vi "KGN Get Limits.vi"(8 "Fehler (Eingang, kein Fehler)":errorcluster, 9 "Info Cluster":T1, 10 "VISA-Ressourcenname":refnum<visa-resource-name>, 11 "device (Eingang)":u32) -> (0 "Fehler (Ausgang)":errorcluster, 1 "Info Cluster out":T1, 2 "VISA-Ressourcenname out":refnum<visa-resource-name>, 3 "dup device (Ausgang)":u32, 4 "Limits Cluster out":cluster{"flow":dbl[], "temp":dbl[]}, 6 "Kommnados gesendet":string)   [LabVIEW 2020, in "Linearisierung v2.lvlib" / "Gasteiler.lvlib" / "HovaCAL_Interface.lvlib" / "KGN.lvlib" / "KGN GUI Get.lvlib"]
uses:
  KGN GUI Get.lvlib
  Controls/Info Cluster.ctl
  get/get.lvlib
  Controls/Controls.lvlib
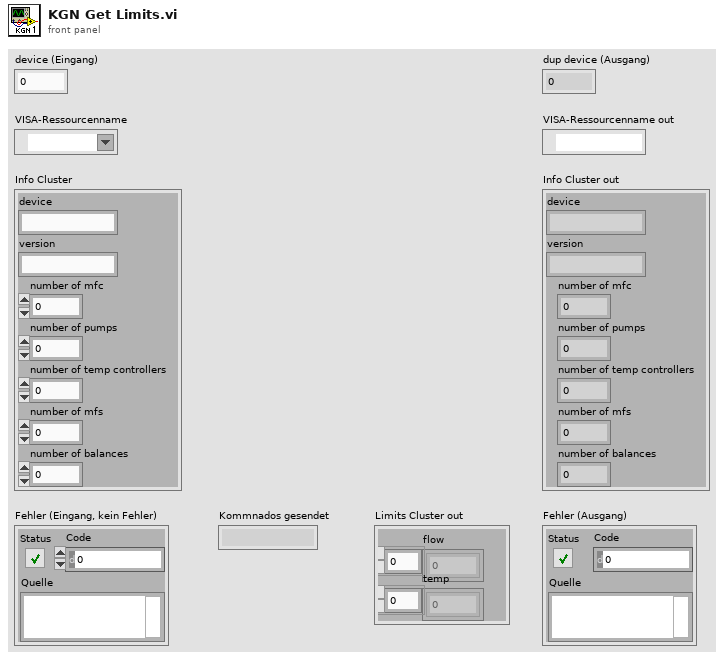
[diagram p1: front panel]
types:
  T1 = typedef "Linearisierung v2.lvlib/Gasteiler.lvlib/HovaCAL_Interface.lvlib/Controls.lvlib/Info Cluster.ctl" = cluster{"device":string, "version":string, "number of mfc":i32, "number of pumps":i32, "number of temp controllers":i32, "number of mfs":i32, "number of balances":i32}
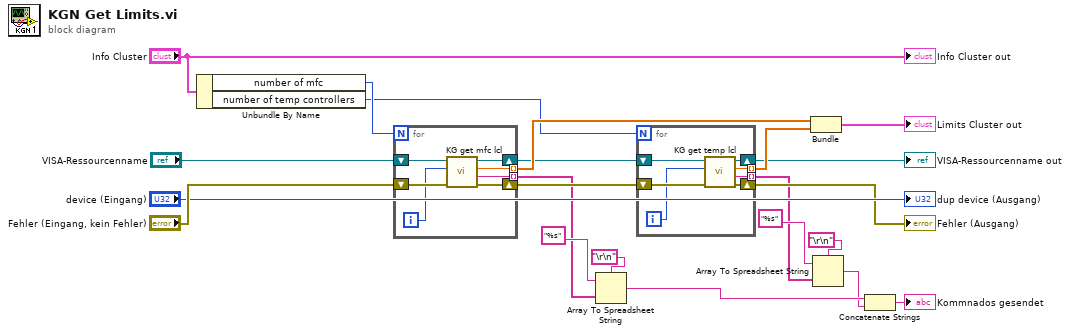
[diagram p0: block diagram]
diagram:
  n1 = Unbundle By Name("Info Cluster") -> ("number of mfc"=w11:i32, "number of temp controllers"=w10:i32)
  n2 = for {
    N: w11 -> [_]
    tunnel: [w28] -> w19 mode=indexing
    shift-right: [w25] -> w14
    shift-left: "Fehler (Eingang, kein Fehler)" -> [w29]
    shift-right: [w26] -> w17
    shift-left: "VISA-Ressourcenname" -> [w27]
    tunnel: [w23] -> w5 mode=indexing
    i -> [w24]
    n3 = call "KG get mfc lcl.vi"("Fehler (Eingang, kein Fehler)"=w29, "mfc"=w24, "VISA-Ressourcenname"=w27) -> ("Fehler (Ausgang)"=w25:errorcluster, "Kommando gesendet"=w23:string, "flow"=w28:dbl, "VISA-Ressourcenname (Ausgang)"=w26:refnum<visa-resource-name>)  [unwired: 5 in]
  }
  n4 = Array To Spreadsheet String(delimiter (Tab)="\r\n", array=w5, 3:"%s" ("Format-String")) -> (spreadsheet string=w3:string)
  n5 = for {
    N: w10 -> [_]
    tunnel: [w35] -> w16 mode=indexing
    shift-right: [w34] -> w15
    shift-left: w17 -> [w36]
    shift-right: [w32] -> w13
    shift-left: w14 -> [w33]
    tunnel: [w30] -> w4 mode=indexing
    i -> [w31]
    n6 = call "KG get temp lcl.vi"("Fehler (Eingang, kein Fehler)"=w33, "controller"=w31, "VISA-Ressourcenname"=w36) -> ("Fehler (Ausgang)"=w32:errorcluster, "Kommando gesendet"=w30:string, "temp"=w35:dbl, "VISA-Ressourcenname (Ausgang)"=w34:refnum<visa-resource-name>)  [unwired: 5 in]
  }
  "Fehler (Ausgang)" <- w13
  "VISA-Ressourcenname out" <- w15
  n7 = Bundle(w19, w16) -> (→"Limits Cluster out":cluster{dbl[], dbl[]})  [unwired: 1 in]
  n8 = Array To Spreadsheet String(delimiter (Tab)="\r\n", array=w4, 3:"%s" ("Format-String")) -> (spreadsheet string=w2:string)
  n9 = Concatenate Strings(w3, w2) -> (→"Kommnados gesendet":string)
  "dup device (Ausgang)" <- "device (Eingang)"
  "Info Cluster out" <- "Info Cluster"
